vi "CD Tree Node Map FGV.vi"(6 "Action":T1, 7 "Parent Name in":string, 8 "error in":errorcluster, 9 "Node Name":string, 10 "Attribute Node":refnum<k20>) -> (0 "error out":errorcluster, 2 "Node Reference":refnum<k20>, 3 "Map Keys":string[](array[string]), 4 "key not found?":bool, 5 "Parent Name out":string)   [LabVIEW 2025]
uses:
  <vilib>/Utility/miscctls.llb/LVMapReplaceAction.ctl
  Types/CD NodeRef Map Action.ctl
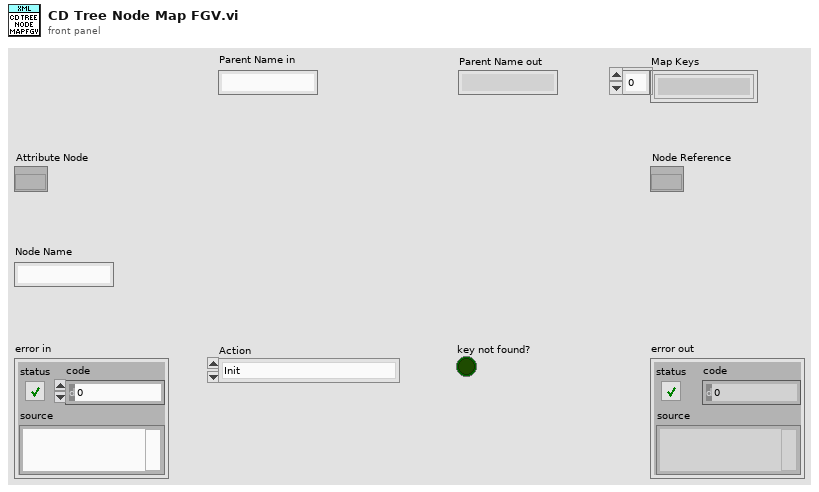
[diagram p1: front panel]
types:
  T1 = typedef "CD NodeRef Map Action.ctl" = enum16{"Init", "Add XMLNodeRef", "Update ParentName", "Delete XMLNodeRef", "Get All Keys", "Get", "skip"}
  T2 = cluster{"Attribute Node":refnum<k20>, "Parent Name":string}
  T3 = typedef "LVMapReplaceAction.ctl" = enum32{"Modify Entry only if found", "Add or Modify Entry", "Delete Entry"}
  T4 = map{string, cluster{"Attribute Node":refnum<k20>, "Parent Name":string}}
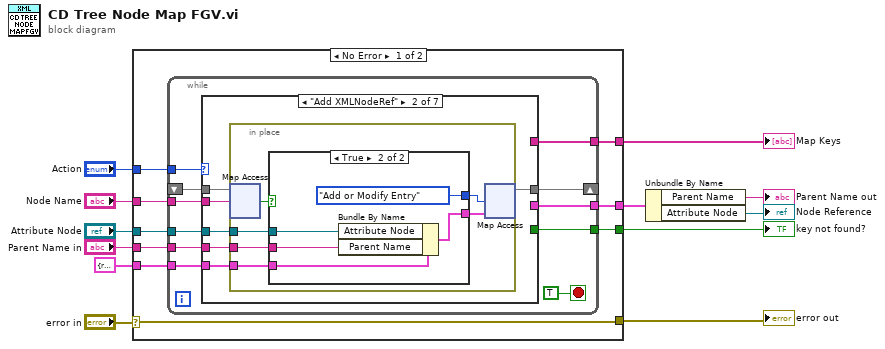
[diagram p0: block diagram]
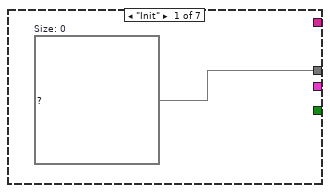
[diagram p2: hidden frame]
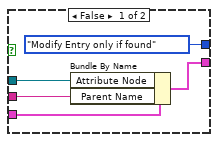
[diagram p3: hidden frame]
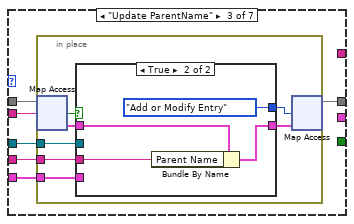
[diagram p4: hidden frame]
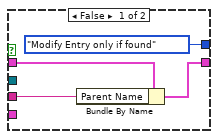
[diagram p5: hidden frame]
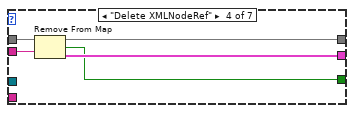
[diagram p6: hidden frame]
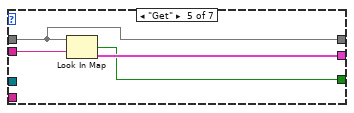
[diagram p7: hidden frame]
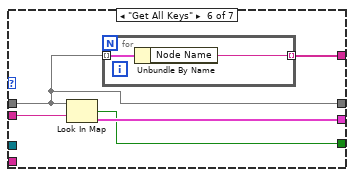
[diagram p8: hidden frame]
diagram:
  n1 = case shown="No Error" "error in" {
    selector: "error in" -> [w18 w94]
    tunnel: "Action" -> [w21 _]
    tunnel: "Node Name" -> [w20 _]
    tunnel: [w19 _] -> w4
    tunnel: [w18 w94] -> w9
    tunnel: "Attribute Node" -> [w17 _]
    tunnel: [w16 _] -> w7
    tunnel: T2 {"Attribute Node"=refnum, "Parent Name"=""} -> [w15 _]
    tunnel: "Parent Name in" -> [w14 _]
    tunnel: [w13 _] -> w1
    frame No Error {
      n2 = while {
        tunnel: w21 -> [w32]
        tunnel: w20 -> [w31]
        tunnel: [w30] -> w19
        tunnel: w17 -> [w29]
        shift-right: [w28] -> _
        shift-left: _ -> [w27]
        tunnel: [w25] -> w16
        tunnel: w15 -> [w24]
        tunnel: w14 -> [w23]
        tunnel: [w22] -> w13
        stop <- TRUE stop-if-true
        n3 = case shown="\"Add XMLNodeRef\"" w32 {
          tunnel: w31 -> [_ w39 w61 w80 w85 w90 _]
          tunnel: [_ _ _ w78 w84 w89 _] -> w30
          tunnel: w29 -> [_ w35 w57 _ _ _ _]
          tunnel: [w33 w38 w60 w79 w82 w87 w93] -> w28
          tunnel: w27 -> [_ w37 w59 w81 w82 w87 w93]
          tunnel: [_ _ _ w77 w83 w88 _] -> w25
          tunnel: w24 -> [_ w36 w58 _ _ _ _]
          tunnel: w23 -> [_ w34 w56 _ _ _ _]
          tunnel: [_ _ _ _ _ w86 _] -> w22
          frame "Init" {
            w33 = T4 {}  # Size: 0
          }
          frame "Add XMLNodeRef" {
            n4 = in-place {
              in-place-border: w35 -> [w43]
              in-place-border: w36 -> [w41]
              in-place-border: w34 -> [w40]
              n5 = in-place-map #1(w37, w39) -> (w45:bool)  [unwired: 1 in, 1 out]
              n6 = case shown="True" w45 {
                tunnel: [w46 w51] -> w42
                tunnel: [LVMapReplaceAction."Modify Entry only if found" ("action") LVMapReplaceAction."Add or Modify Entry" ("action")] -> w44
                tunnel: w43 -> [w47 w52]
                tunnel: w41 -> [w49 w54]
                tunnel: w40 -> [w48 w53]
                frame False {
                  n7 = Bundle By Name(cluster=w49, "Attribute Node"=w47, "Parent Name"=w48) -> (w46:T2)
                }
                frame True {
                  n8 = Bundle By Name(cluster=w54, "Attribute Node"=w52, "Parent Name"=w53) -> (w51:T2)
                }
              }
              n9 = in-place-map #1(w42, w44) -> (w38:T4)  [unwired: 2 out]
            }
          }
          frame "Update ParentName" {
            n10 = in-place {
              in-place-border: w57 -> [w66]
              in-place-border: w58 -> [w64]
              in-place-border: w56 -> [w63]
              n11 = in-place-map #2(w59, w61) -> (w62:T2, w68:bool)  [unwired: 1 in]
              n12 = case shown="True" w68 {
                tunnel: [w70 w74] -> w65
                tunnel: [LVMapReplaceAction."Modify Entry only if found" ("action") LVMapReplaceAction."Add or Modify Entry" ("action")] -> w67
                tunnel: w66 -> [_ _]
                tunnel: w64 -> [_ _]
                tunnel: w63 -> [w71 w75]
                tunnel: w62 -> [w69 w73]
                frame False {
                  n13 = Bundle By Name(cluster=w69, "Parent Name"=w71) -> (w70:T2)
                }
                frame True {
                  n14 = Bundle By Name(cluster=w73, "Parent Name"=w75) -> (w74:T2)
                }
              }
              n15 = in-place-map #2(w65, w67) -> (w60:T4)  [unwired: 2 out]
            }
          }
          frame "Delete XMLNodeRef" {
            n16 = Remove From Map(10:w80, 11:w81) -> (1:w78:T2, 2:w77:bool, 3:w79:T4)
          }
          frame "Get" {
            n17 = Look In Map(map=w82, key=w85) -> (key not found?=w83:bool, value=w84:T2)  [unwired: 1 in]
          }
          frame "Get All Keys" {
            n18 = Look In Map(map=w87, key=w90) -> (key not found?=w88:bool, value=w89:T2)  [unwired: 1 in]
            n19 = for {
              tunnel: w87 -> [w92] mode=indexing
              tunnel: [w91] -> w86 mode=indexing
              n20 = Unbundle By Name(w92) -> ("Node Name"=w91:string)
            }
          }
          frame "skip" {
          }
        }
      }
    }
    frame Error {
    }
  }
  "error out" <- w9
  "key not found?" <- w7
  "Map Keys" <- w1
  n21 = Unbundle By Name(w4) -> ("Parent Name"=→"Parent Name out":string, "Attribute Node"=→"Node Reference":refnum<k20>)
